vi "Get Data.vi"(8 "error in":errorcluster, 11 "cPAS in":refnum<class "cPAS.lvclass">) -> (0 "error out":errorcluster, 3 "cPAS out":refnum<class "cPAS.lvclass">)   [LabVIEW 2015, in "cPAS.lvclass"]
doc: "Retrieve data from the photoacoustic data acquisition system. In the current configuration, this includes housekeeping data such as temperatures, relative humidities and etc. as well as the high frequency data from the speakers and photodiodes.\n\nTODO: The serial acquisition has to be included as well as un-hardcoding the acquisition time."
uses:
  cPAS.lvclass
  Devices/Alicat/Session Based/Data/Alicat Data.lvclass
  cPAS.lvclass/cPAS.ctl
  Data/cPAS Data.lvclass
  Reusable/General/Temperature/Thermistor Config.ctl
  Reusable/General/Temperature/Thermistor Position.ctl
  Controls/Flags.ctl
  Data/cPAS Data.lvclass/cPAS Data.ctl
  <vilib>/DAQmx/read.llb/DAQmx Read (Analog 2D DBL NChan NSamp).vi
  <vilib>/DAQmx/read.llb/DAQmx Read (Analog 2D I16 NChan NSamp).vi
  <vilib>/Analysis/baseanly.llb/Mean (DBL).vi
  Data/Write Serial Data.vi
  Read Acoustic.vi
  Read Housekeeping.vi
  Reusable/PAS/Main/Write goodData.vi
  Reusable/PAS/Main/Read Data.vi
  Read Serial IO.vi
  <vilib>/DAQmx/miscellaneous.llb/DAQmx Fill In Error Info.vi
  Reusable/Data/Write measTime.vi
  Data/Write Thum.vi
  Data/Write dcVolts.vi
  Reusable/PAS/Data/Main/Write filter.vi
  Reusable/PAS/Data/Main/Write O3 flag.vi
  Reusable/PAS/Data/Main/Write Current Cell.vi
  Reusable/PAS/Data/Main/Write Cell Microphone Signal.vi
  Reusable/PAS/Data/Main/Write Cell Laser Diode Signal.vi
  Reusable/PAS/Data/Main/Write Cell Housekeeping.vi
  Data/Write Cell T2.vi
  Reusable/PAS/Main/Write Data.vi
  Reusable/PAS/Data/Main/PAS Data.lvclass
  Devices/Configurable Device/Configurable Device.lvclass
  Reusable/Instrument/Instrument.lvclass
  <resource>/objmgr/daqmx.rc
  Reusable/General/Temperature/Temperature.lvlib
  <vilib>/Analysis/NI_AALBase.lvlib
panel:
  out "Array":refnum<class "Alicat Data.lvclass">[](array[class])
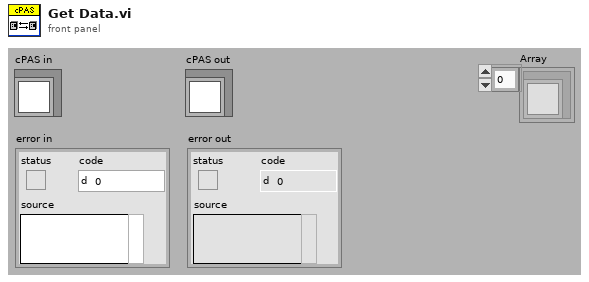
[diagram p1: front panel]
types:
  T1 = typedef "Flags.ctl" = enum8{"Autospeaker", "Link cycles", "Autofilter", "O3 Cal", "Filter Position"}
  T2 = typedef "Temperature.lvlib/Thermistor Position.ctl" = enum8{"Bottom", "Top"}
  T3 = typedef "Temperature.lvlib/Thermistor Config.ctl" = cluster{"Vsource":dbl, "SH Coeff":dbl[], "R1":dbl, "Rref":dbl[], "Tref":dbl[]}
  T4 = cluster{"[0]":sgl, "[1]":sgl, "[2]":sgl, "[3]":sgl, "[4]":sgl}
  T5 = cluster{"[0]":sgl, "[1]":sgl, "[2]":sgl, "[3]":sgl}
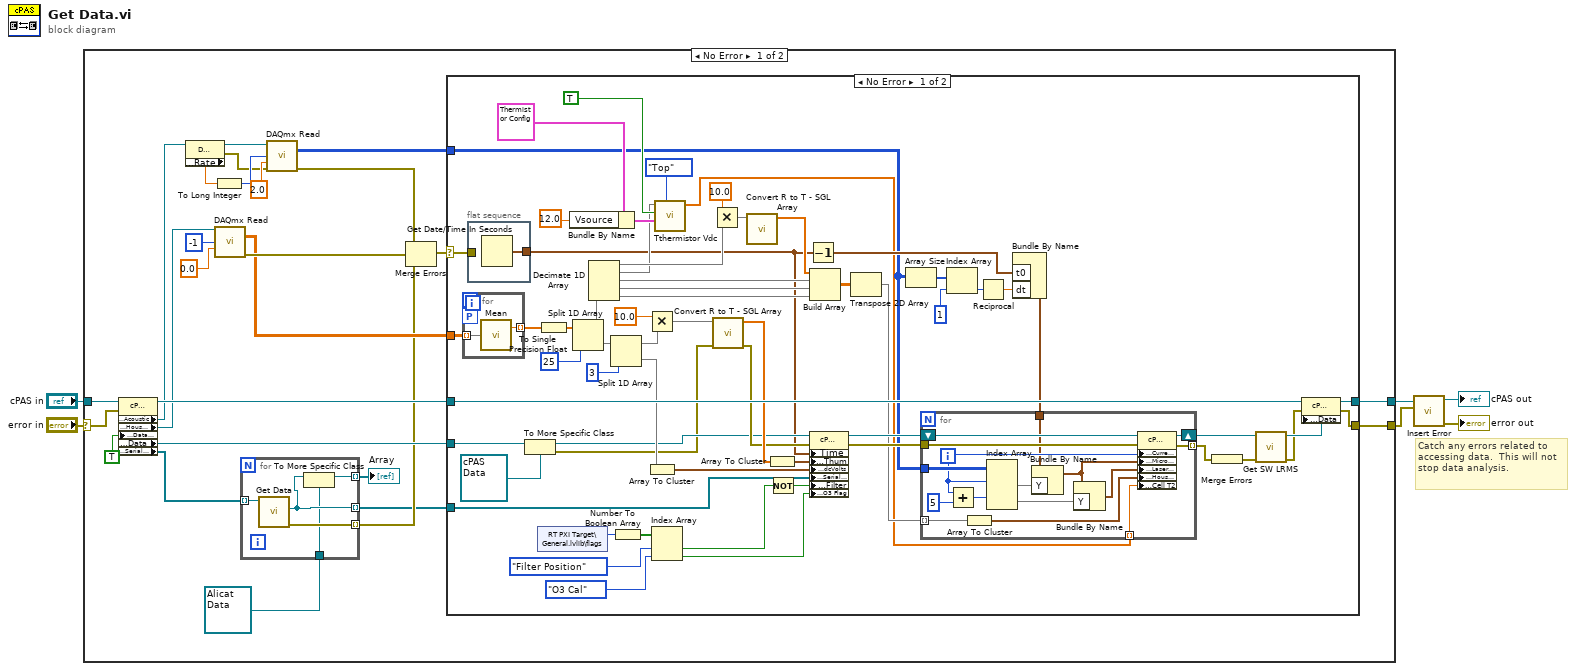
[diagram p0: block diagram]
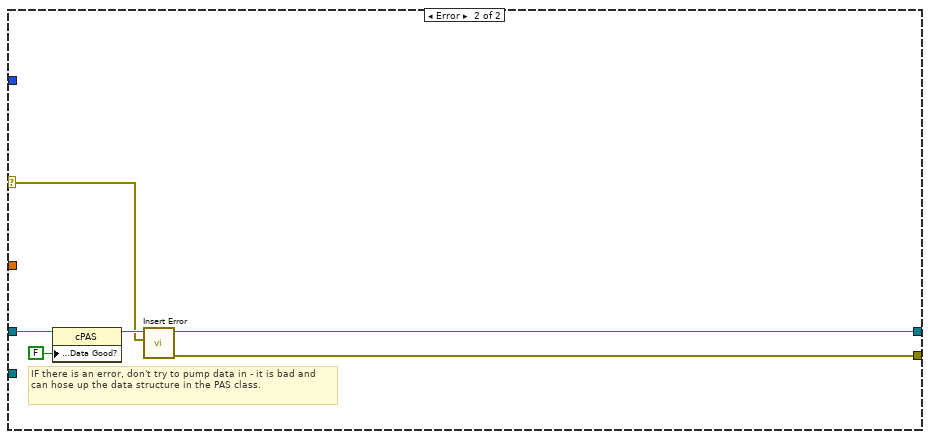
[diagram p2: hidden frame]
diagram:
  # "Catch any errors related to accessing data.  This will not stop data analysis."
  n1 = case shown="No Error" "error in" {
    selector: "error in" -> [w21 w126]
    tunnel: [w30 w126] -> w2
    tunnel: [w31 w125] -> w4
    tunnel: "cPAS in" -> [w22 w125]
    frame No Error {
      n2 = property class="cPAS"(reference=w22, error in=w21, "Data Access:Data Good?"=TRUE ("goodData")) -> (reference out=w19:refnum<class "cPAS.lvclass">, "Accessors:Acoustic"=w13:refnum<k21>, "Accessors:Housekeeping"=w12:refnum<k21>, "Data Access:Data"=w16:refnum<class "PAS Data.lvclass">, "Data Access:Serial IO"=w11:refnum<class "Configurable Device.lvclass">[])  [unwired: 1 out]
      n3 = property class="DAQmx Timing"(reference=w13) -> (reference out=w27:refnum<k21>, error out=w26:errorcluster, "SampClk.Rate"=w25:dbl)  [unwired: 1 in]
      n4 = To Long Integer(number=w25) -> (32bit integer=w29:i32)
      n5 = call-poly <vilib>:"DAQmx Read.vi"("task/channels in"=w12, "number of samples per channel"=-1, "timeout"=0.0) -> ("data"=w15:dbl[][], "error out"=w32:errorcluster)  [unwired: 10 in, 1 out]
      n6 = for {
        tunnel: w11 -> [w37] mode=indexing
        tunnel: [w35] -> w9 mode=indexing
        tunnel: [w36] -> w10 mode=indexing
        tunnel: [w34] -> w7 mode=indexing
        tunnel: refnum<class "Alicat Data.lvclass"> refnum ("Alicat Data in") -> [w33]
        n7 = call-dynamic "Get Data.vi"("Cfg Dev in"=w37) -> ("error out"=w36:errorcluster, "Base Data Lib:Data"=w35:refnum<class "Data.lvclass">)  [unwired: 8 in, 1 out]
        n8 = To More Specific Class(target class=w33, reference=w35) -> (specific class reference=w34:refnum<class "Alicat Data.lvclass">)  [unwired: 1 in, 1 out]
      }
      "Array" <- w7
      n9 = call-poly <vilib>:"DAQmx Read.vi"("task/channels in"=w27, "number of samples per channel"=w29, "timeout"=2.0, "error in"=w26) -> ("data"=w18:i16[][], "error out"=w14:errorcluster)  [unwired: 9 in, 1 out]
      n10 = Merge Errors(w14, w32, w10) -> (w17:errorcluster)
      n11 = case shown="No Error" w17 {
        selector: w17 -> [w50 w120]
        tunnel: [w96 w124] -> w31
        tunnel: [w95 w123] -> w30
        tunnel: w16 -> [w77 _]
        tunnel: w19 -> [w94 w122]
        tunnel: w15 -> [w74 _]
        tunnel: w18 -> [w56 _]
        tunnel: w9 -> [w73 _]
        frame No Error {
          n12 = for {
            tunnel: w74 -> [w102] mode=indexing
            tunnel: [w101] -> w75 mode=indexing
            workers-P: _ -> [_]
            n13 = call-poly <vilib>:"Mean.vi"("X"=w102) -> ("mean"=w101:dbl)  [unwired: 1 out]
          }
          n14 = flat-sequence {
            tunnel: [w100] -> w58
            tunnel: w50 -> [_]
            frame #0 {
              n15 = Get Date/Time In Seconds() -> (seconds since 1Jan1904=w100:timestamp)
            }
          }
          n16 = To More Specific Class(target class=refnum<class "cPAS Data.lvclass"> refnum ("cPAS Data"), reference=w77) -> (specific class reference=w76:refnum<class "cPAS Data.lvclass">, error out=w59:errorcluster)  [unwired: 1 in]
          n17 = shared-variable "RT PXI Target\\General.lvlib\\flags"() -> (w44:u8)  [unwired: 1 in, 1 out]
          n18 = To Single Precision Float(number=w75) -> (single precision float=w90:sgl[])
          n19 = Bundle By Name(cluster=T3 {"Vsource"=10.0, "SH Coeff"=[0.0010291947674223878, 0.00023912751839781632, 1.5662771497033316e-07], "R1"=10.0, "Rref"=[], "Tref"=[]} ("thermCirc"), "Vsource"=12.0) -> (w63:T3)
          n20 = Split 1D Array(array=w90, index=25) -> (first subarray=w85:sgl[], second subarray=w83:sgl[])
          n21 = Decimate 1D Array(w85) -> (w72:sgl[], w61:sgl[], w86:sgl[], w87:sgl[], w79:sgl[])
          n22 = Split 1D Array(array=w83, index=3) -> (first subarray=w68:sgl[], second subarray=w81:sgl[])
          n23 = Number To Boolean Array(number=w44) -> (Boolean array=w43:bool[])
          n24 = Multiply(x=sgl 10.0, y=w68) -> (x*y=w67:sgl[])
          n25 = Array To Cluster(array=w81) -> (cluster=w80:T4)
          n26 = Index Array(array=w43, index #1=Flags."Filter Position" ("Flags"), index #2=Flags."O3 Cal" ("Flags")) -> (element #1=w39:bool, element #2=w42:bool)
          n27 = call "Tthermistor Vdc.vi"("ThermConfig"=Thermistor_Position."Top", "thermCirc"=w63, "Init"=TRUE, "Vdc"=w61) -> ("T"=w49:dbl[])  [unwired: 4 in, 1 out]
          n28 = Multiply(x=sgl 10.0 ("mean"), y=w72) -> (x*y=w70:sgl[])
          n29 = call "Convert R to T - SGL Array.vi"("error in"=w59, "R"=w67) -> ("error out"=w82:errorcluster, "T"=w92:sgl[])  [unwired: 8 in]
          n30 = call "Convert R to T - SGL Array.vi"("R"=w70) -> ("T"=w69:sgl[])  [unwired: 9 in, 1 out]
          n31 = Array To Cluster(array=w92) -> (cluster=w91:cluster{"T[0]":sgl, "T[1]":sgl})
          n32 = Not(x=w39) -> (.not. x?=w38:bool)
          n33 = Decrement(x=w58) -> (x-1=w57:timestamp)
          n34 = Build Array(w69, w86, w87, w79) -> (w88:sgl[][])
          n35 = property class="cPAS Data"(reference=w76, error in=w82, "Time"=w58, "Accessors:Thum"=w91, "Accessors:dcVolts"=w80, "Accessors:Serial Data"=w73, "Data Access:Filter"=w38, "Data Access:O3 Flag"=w42) -> (reference out=w98:refnum<class "cPAS Data.lvclass">, error out=w97:errorcluster)
          n36 = Transpose 2D Array(2D array=w88) -> (transposed array=w84:sgl[][])
          n37 = Array Size(array=w56) -> (size(s)=w55:i32[])
          n38 = Index Array(array=w55, index=1) -> (element=w53:i32)
          n39 = Reciprocal(x=w53) -> (1/x=w52:dbl)
          n40 = Bundle By Name("t0"=w57, "dt"=w52) -> (w51:waveform(i16))  [unwired: 1 in]
          n41 = for {
            shift-right: [w117] -> w48
            shift-left: w98 -> [w118]
            tunnel: [w116] -> w99 mode=indexing
            tunnel: w97 -> [w115]
            tunnel: w56 -> [w114]
            tunnel: w84 -> [w112] mode=indexing
            tunnel: w51 -> [w108]
            tunnel: w49 -> [w103] mode=indexing
            i -> [w111]
            n42 = Add(x=w111, y=5) -> (x+y=w107:i32)
            n43 = Array To Cluster(array=w112) -> (cluster=w113:T5)
            n44 = Index Array(array=w114, index (row) #1=w111, index (row) #2=w107) -> (element #1=w109:i16[], element #2=w104:i16[])  [unwired: 2 in]
            n45 = Bundle By Name(cluster=w108, "Y"=w109) -> (w106:waveform(i16))
            n46 = Bundle By Name(cluster=w106, "Y"=w104) -> (w105:waveform(i16))
            n47 = property class="cPAS Data"(reference=w118, error in=w115, "Data Access:Current Cell"=w111, "Data Access:Microphone"=w106, "Data Access:Laser Diode"=w105, "Data Access:Housekeeping"=w113, "Accessors:Cell T2"=w103) -> (reference out=w117:refnum<class "cPAS Data.lvclass">, error out=w116:errorcluster)
          }
          n48 = Merge Errors(w99) -> (w46:errorcluster)
          n49 = call "Get SW LRMS.vi"("error in"=w46, "cPAS Data in"=w48) -> ("error out"=w45:errorcluster, "cPAS Data out"=w47:refnum<class "cPAS Data.lvclass">)  [unwired: 8 in]
          n50 = property class="cPAS"(reference=w94, error in=w45, "Data Access:Data"=w47) -> (reference out=w96:refnum<class "cPAS.lvclass">, error out=w95:errorcluster)
        }
        frame Error {
          # "IF there is an error, don't try to pump data in - it is bad and can hose up the data structure in the PAS class."
          n51 = property class="cPAS"(reference=w122, "Data Access:Data Good?"=FALSE ("Data Good?")) -> (reference out=w121:refnum<class "cPAS.lvclass">)  [unwired: 1 in, 1 out]
          n52 = call "Insert Error.vi"("err"=w120, "Instrument in"=w121) -> ("error out"=w123:errorcluster, "Instrument out"=w124:refnum<class "cPAS.lvclass">)  [unwired: 7 in, 1 out]
        }
      }
    }
    frame Error {
    }
  }
  n53 = call "Insert Error.vi"("err"=w2, "Instrument in"=w4) -> ("error out"=→"error out":errorcluster, "Instrument out"=→"cPAS out":refnum<class "cPAS.lvclass">)  [unwired: 7 in, 1 out]
